vi "CALC_TRAN_TIME_IMP_WIDT.vi"(0 "VISA IN":refnum<visa-resource-name>, 1 "Impulse Width(sec)":i32, 5 "error in":errorcluster, 7 "Channel":i32) -> (14 "VISA Out":refnum<visa-resource-name>, 19 "error out":errorcluster)   [LabVIEW 2018, in "PNA-X.lvlib"]
doc: "CALCulate<cnum>:TRANsform:TIME:IMPulse:WIDTh <num> \n(Read-Write) Sets the impulse width for the transform window. \nSee Critical Note \nParameters \n<cnum> Channel number of the measurement. There must be a selected measurement \non that channel. If unspecified, <cnum> is set to 1. \n<num> Impulse width in seconds; Choose any number between: \n.6 / frequency span and 1.39 / frequency span \nExamples CALC:TRAN:TIME:IMP:WIDTh 10 \ncalculate2:transform:time:impulse:width 13 \nQuery Syntax CALCulate<cnum>:TRANsform:TIME:IMPulse:WIDTh? \nReturn Type Numeric \nDefault .98 / Default Span"
uses:
  PNA-X.lvlib
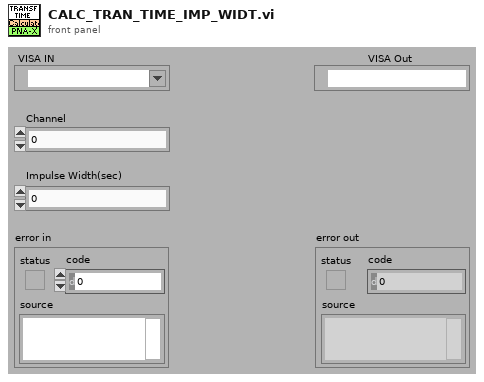
[diagram p1: front panel]
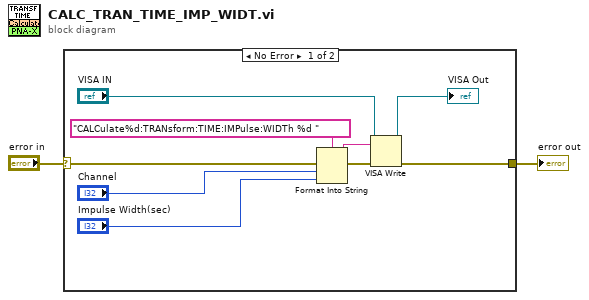
[diagram p0: block diagram]
diagram:
  n1 = case shown="No Error" "error in" {
    selector: "error in" -> [w11 w12]
    tunnel: [w6 w12] -> w1
    frame No Error {
      n2 = Format Into String(format string="CALCulate%d:TRANsform:TIME:IMPulse:WIDTh %d " ("Cmdline"), error in=w11, "Channel", "Impulse Width(sec)") -> (resulting string=w9:string, error out=w10:errorcluster)  [unwired: 1 in]
      n3 = VISA Write(VISA resource name="VISA IN", write buffer=w9, error in (no error)=w10) -> (VISA resource name out=→"VISA Out":refnum<visa-resource-name>, error out=w6:errorcluster)  [unwired: 1 out]
    }
    frame Error {
    }
  }
  "error out" <- w1
